vi "makeDecisions.vi"(8 "error in (no error)":errorcluster, 10 "model":refnum<class "Model.lvclass">, 11 "EndingCycleState in":refnum<class "EndingCycleState.lvclass">) -> (0 "error out":errorcluster, 2 "model 2":refnum<class "Model.lvclass">, 3 "EndingCycleState out":refnum<class "EndingCycleState.lvclass">)   [LabVIEW 2013, in "EndingCycleState.lvclass"]
uses:
  EndingCycleState.lvclass
  Model/Model/Model.lvclass
  AutomatedMotionState/AutomatedMotionState.lvclass
  Typedefs/StateSelector.ctl
  Typedefs/M2AADTTypedefs.lvlib
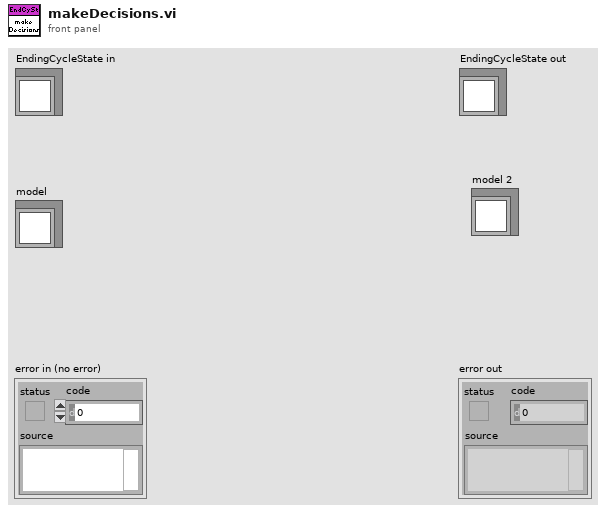
[diagram p1: front panel]
types:
  T1 = typedef "M2AADTTypedefs.lvlib/StateSelector.ctl" = enum16{"EndingCycleState", "FaultState", "InteractiveMotionState", "MovingToNewForceState", "OffState", "PausingState", "StandbyState", "StoppedState"}
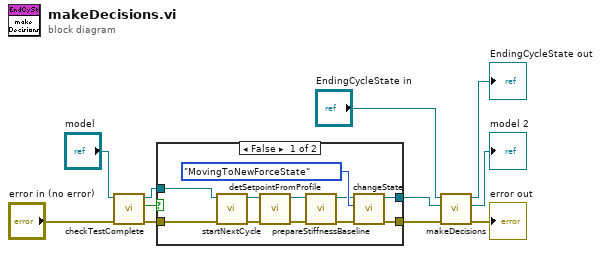
[diagram p0: block diagram]
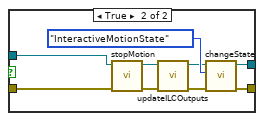
[diagram p2: hidden frame]
diagram:
  n1 = call "checkTestComplete.vi"("error in (no error)"="error in (no error)", "Model in"="model") -> ("error out"=w4:errorcluster, "testCompleteIsTrue"=w1:bool, "Model out"=w6:refnum<class "Model.lvclass">)  [unwired: 7 in]
  n2 = case shown="False" w1 {
    tunnel: w6 -> [w22 w31]
    tunnel: w4 -> [w20 w29]
    tunnel: [w19 w28] -> w3
    tunnel: [w21 w27] -> w2
    frame False {
      n3 = call "startNextCycle.vi"("error in (no error)"=w20, "Model in"=w22) -> ("error out"=w16:errorcluster, "Model out"=w17:refnum<class "Model.lvclass">)  [unwired: 8 in]
      n4 = call "detSetpointFromProfile.vi"("error in (no error)"=w16, "Model in"=w17) -> ("error out"=w13:errorcluster, "Model out"=w15:refnum<class "Model.lvclass">)  [unwired: 8 in]
      n5 = call "prepareStiffnessBaseline.vi"("error in (no error)"=w13, "Model in"=w15) -> ("error out"=w12:errorcluster, "Model out"=w14:refnum<class "Model.lvclass">)  [unwired: 8 in]
      n6 = call "changeState.vi"("error in (no error)"=w12, "State:"=StateSelector."MovingToNewForceState", "Model in"=w14) -> ("error out"=w19:errorcluster, "Model out"=w21:refnum<class "Model.lvclass">)  [unwired: 7 in]
    }
    frame True {
      n7 = call "stopMotion.vi"("error in (no error)"=w29, "Model in"=w31) -> ("error out"=w25:errorcluster, "Model out"=w26:refnum<class "Model.lvclass">)  [unwired: 8 in]
      n8 = call "updateILCOutputs.vi"("error in (no error)"=w25, "Model in"=w26) -> ("error out"=w23:errorcluster, "Model out"=w24:refnum<class "Model.lvclass">)  [unwired: 8 in]
      n9 = call "changeState.vi"("error in (no error)"=w23, "State:"=StateSelector."InteractiveMotionState", "Model in"=w24) -> ("error out"=w28:errorcluster, "Model out"=w27:refnum<class "Model.lvclass">)  [unwired: 7 in]
    }
  }
  n10 = call-parent "makeDecisions.vi"("error in (no error)"=w3, "model"=w2, "EnabledState in"="EndingCycleState in") -> ("error out"=→"error out":errorcluster, "model 2"=→"model 2":refnum<class "Model.lvclass">, "EnabledState out"=→"EndingCycleState out":refnum<class "EndingCycleState.lvclass">)  [unwired: 6 in]
